vi "Spark MAX_Extract out all Parameter Data.vi"(11 "MotorControlDeviceRef":T4={"DeviceStatus"={"status"=FALSE, "code"=0, "source"=""}, "Type"=enum."CAN", "PWM"={"PWM Channel"=enum."Invalid", "DeadBand"={"Name"="", "maxPositivePwm"=0, "minPositivePwm"=0, "centerPwm"=0, "maxNegativePwm"=0, "minNegativePwm"=0, "angularRange"=0}}, "CAN"={"Device Number"=8, "SetOutput VI Ref"=variant, "GetOutput VI Ref"=variant, "Enable VI Ref"=variant, "Disable VI Ref"=variant, "Data"=variant(cluster{"Ext ID":u32, "Motor Type":enum16{"Brushed", "Brushless"}} {"Ext ID"=33882120, "Motor Type"=enum."Brushed"})}, "Invert"=FALSE, "DIO PWM"={"PWM \"Enable\" Channel"=enum."Invalid", "DIOChannel"=enum."Invalid", "PWM Rate"=0.0}}) -> (0 "Error Out":errorcluster, 1 "Type Out":T3, 2 "Raw Parameter Out":u32, 3 "MotorControlDeviceRef Out":T4={"DeviceStatus"={"status"=FALSE, "code"=0, "source"=""}, "Type"=enum."CAN", "PWM"={"PWM Channel"=enum."Invalid", "DeadBand"={"Name"="", "maxPositivePwm"=0, "minPositivePwm"=0, "centerPwm"=0, "maxNegativePwm"=0, "minNegativePwm"=0, "angularRange"=0}}, "CAN"={"Device Number"=8, "SetOutput VI Ref"=variant, "GetOutput VI Ref"=variant, "Enable VI Ref"=variant, "Disable VI Ref"=variant, "Data"=variant(cluster{"Ext ID":u32, "Motor Type":enum16{"Brushed", "Brushless"}} {"Ext ID"=33882120, "Motor Type"=enum."Brushed"})}, "Invert"=FALSE, "DIO PWM"={"PWM \"Enable\" Channel"=enum."Invalid", "DIOChannel"=enum."Invalid", "PWM Rate"=0.0}}, 5 "Array Out":T1[](array[typedef]) {"Float" format="%#_4f"})   [LabVIEW 2020]
uses:
  <vilib>/Rock Robotics/WPI/MotorControl/WPI_MotorControlDeviceRef.ctl
  <vilib>/Rock Robotics/WPI/MotorControl/WPI_MotorControlType.ctl
  <vilib>/Rock Robotics/SystemInterfaces/DIO/FPGA_DIOPWMChannel.ctl
  <vilib>/Rock Robotics/WPI/PWM/WPI_PWMDeadband.ctl
  <vilib>/Rock Robotics/SystemInterfaces/DIO/FPGA_DIOChannel.ctl
  <vilib>/Rock Robotics/WPI/ThirdParty/REV Robotics/REVLib/Typedef/Spark MAX Parameter Type.ctl
  Cluster_Spark Max parameter data.ctl
  <vilib>/Rock Robotics/WPI/ThirdParty/REV Robotics/REVLib/Typedef/Spark MAX Parameter ID.ctl
  <vilib>/Rock Robotics/WPI/ThirdParty/REV Robotics/REVLib/Typedef/Spark MAX Variant Data.ctl
  7c812163-354c-4a87-889c-090e08b6996c.vi
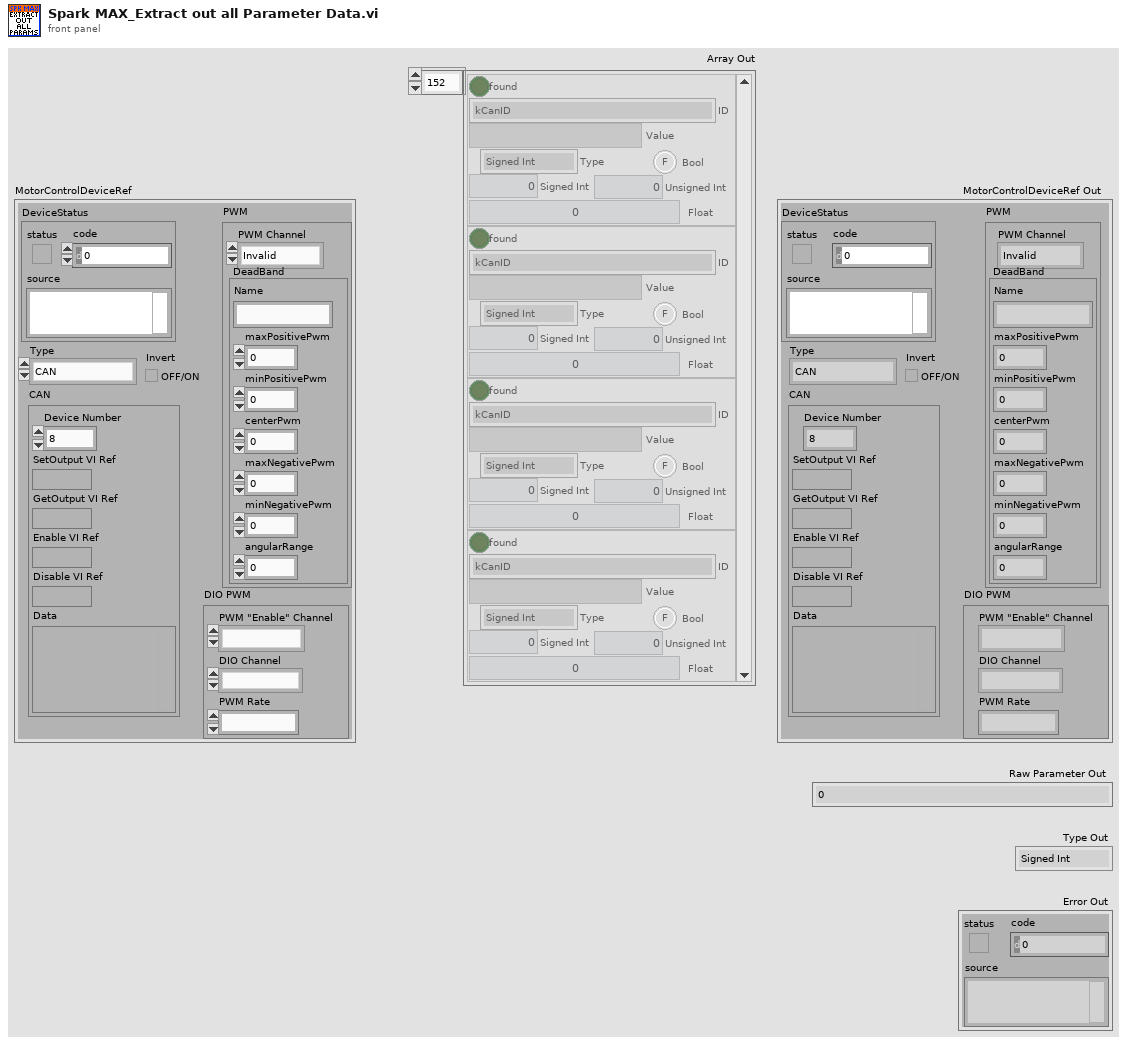
[diagram p1: front panel]
types:
  T1 = typedef "Cluster_Spark Max parameter data.ctl" = cluster{"found":bool, "ID":T2, "Value":string, "Type":T3, "Signed Int":i32, "Unsigned Int":u32, "Float":dbl, "Bool":bool}
  T2 = typedef "Spark MAX Parameter ID.ctl" = enum16{"kCanID", "kInputMode", "kMotorType", "kCommAdvance", "kSensorType", "kCtrlType", "kIdleMode", "kInputDeadband", "kFeedbackSensorPID0", "kFeedbackSensorPID1", "kPolePairs", "kCurrentChop", "kCurrentChopCycles", "kP_0", "kI_0", "kD_0", "kF_0", "kIZone_0", "kDFilter_0", "kOutputMin_0", "kOutputMax_0", "kP_1", "kI_1", "kD_1", "kF_1", "kIZone_1", "kDFilter_1", "kOutputMin_1", "kOutputMax_1", "kP_2", "kI_2", "kD_2", "kF_2", "kIZone_2", "kDFilter_2", "kOutputMin_2", "kOutputMax_2", "kP_3", "kI_3", "kD_3", "kF_3", "kIZone_3", "kDFilter_3", "kOutputMin_3", "kOutputMax_3", "kInverted", "kOutputRatio", "kSerialNumberLow", "kSerialNumberMid", "kSerialNumberHigh", "kLimitSwitchFwdPolarity", "kLimitSwitchRevPolarity", "kHardLimitFwdEn", "kHardLimitRevEn", "kSoftLimitFwdEn", "kSoftLimitRevEn", "kRampRate", "kFollowerID", "kFollowerConfig", "kSmartCurrentStallLimit", "kSmartCurrentFreeLimit", "kSmartCurrentConfig", "kSmartCurrentReserved", "kMotorKv", "kMotorR", "kMotorL", "kMotorRsvd1", "kMotorRsvd2", "kMotorRsvd3", "kEncoderCountsPerRev", "kEncoderAverageDepth", "kEncoderSampleDelta", "kEncoderInverted", "kEncoderRsvd1", "kClosedLoopVoltageMode", "kCompensatedNominalVoltage", "kSmartMotionMaxVelocity_0", "kSmartMotionMaxAccel_0", "kSmartMotionMinVelOutput_0", "kSmartMotionAllowedClosedLoopError_0", "kSmartMotionAccelStrategy_0", "kSmartMotionMaxVelocity_1", "kSmartMotionMaxAccel_1", "kSmartMotionMinVelOutput_1", "kSmartMotionAllowedClosedLoopError_1", "kSmartMotionAccelStrategy_1", "kSmartMotionMaxVelocity_2", "kSmartMotionMaxAccel_2", "kSmartMotionMinVelOutput_2", "kSmartMotionAllowedClosedLoopError_2", "kSmartMotionAccelStrategy_2", "kSmartMotionMaxVelocity_3", "kSmartMotionMaxAccel_3", "kSmartMotionMinVelOutput_3", "kSmartMotionAllowedClosedLoopError_3", "kSmartMotionAccelStrategy_3", "kIMaxAccum_0", "kSlot3Placeholder1_0", "kSlot3Placeholder2_0", "kSlot3Placeholder3_0", "kIMaxAccum_1", "kSlot3Placeholder1_1", "kSlot3Placeholder2_1", "kSlot3Placeholder3_1", "kIMaxAccum_2", "kSlot3Placeholder1_2", "kSlot3Placeholder2_2", "kSlot3Placeholder3_2", "kIMaxAccum_3", "kSlot3Placeholder1_3", "kSlot3Placeholder2_3", "kSlot3Placeholder3_3", "kPositionConversionFactor", "kVelocityConversionFactor", "kClosedLoopRampRate", "kSoftLimitFwd", "kSoftLimitRev", "kSoftLimitRsvd0", "kSoftLimitRsvd1", "kAnalogPositionConversion", "kAnalogVelocityConversion", "kAnalogAverageDepth", "kAnalogSensorMode", "kAnalogInverted", "kAnalogSampleDelta", "kAnalogRsvd0", "kAnalogRsvd1", "kDataPortConfig", "kAltEncoderCountsPerRev", "kAltEncoderAverageDepth", "kAltEncoderSampleDelta", "kAltEncoderInverted", "kAltEncoderPositionConversion", "kAltEncoderVelocityConversion", "kAltEncoderRsvd0", "kAltEncoderRsvd1", "kHallSensorSampleRate", "kHallSensorAverageDepth", "kNumParameters", "kDutyCyclePositionFactor", "kDutyCycleVelocityFactor", "kDutyCycleInverted", "kDutyCycleSensorMode", "kDutyCycleAverageDepth", "kDutyCycleSampleDelta", "kDutyCycleOffsetv1p6p2", "kDutyCycleRsvd0", "kDutyCycleRsvd1", "kDutyCycleRsvd2", "kPositionPIDWrapEnable", "kPositionPIDMinInput", "kPositionPIDMaxInput", "kDutyCycleZeroCentered", "kDutyCyclePrescalar", "kDutyCycleOffset"}
  T3 = typedef "Spark MAX Parameter Type.ctl" = enum16{"Signed Int", "Unsigned Int", "Float", "Bool"}
  T4 = typedef "WPI_MotorControlDeviceRef.ctl" = cluster{"DeviceStatus":errorcluster, "Type":T5, "PWM":cluster{"PWM Channel":T6, "DeadBand":T7}, "CAN":cluster{"Device Number":u8, "SetOutput VI Ref":variant, "GetOutput VI Ref":variant, "Enable VI Ref":variant, "Disable VI Ref":variant, "Data":variant}, "Invert":bool, "DIO PWM":cluster{"PWM \"Enable\" Channel":T6, "DIOChannel":T8, "PWM Rate":dbl}}
  T5 = typedef "WPI_MotorControlType.ctl" = enum16{"PWM", "CAN", "DIO PWM"}
  T6 = typedef "FPGA_DIOPWMChannel.ctl" = enum8{"PWM 0", "PWM 1", "PWM 2", "PWM 3", "PWM 4", "PWM 5", "PWM 6", "PWM 7", "PWM 8", "PWM 9", "PWM MXP 0", "PWM MXP 1", "PWM MXP 2", "PWM MXP 3", "PWM MXP 4", "PWM MXP 5", "PWM MXP 6", "PWM MXP 7", "PWM MXP 8", "PWM MXP 9", "Invalid"}
  T7 = typedef "WPI_PWMDeadband.ctl" = cluster{"Name":string, "maxPositivePwm":i32, "minPositivePwm":i32, "centerPwm":i32, "maxNegativePwm":i32, "minNegativePwm":i32, "angularRange":u16}
  T8 = typedef "FPGA_DIOChannel.ctl" = enum8{"DIO 0", "DIO 1", "DIO 2", "DIO 3", "DIO 4", "DIO 5", "DIO 6", "DIO 7", "DIO 8", "DIO 9", "DIO MXP 0", "DIO MXP 1", "DIO MXP 2", "DIO MXP 3", "DIO MXP 4", "DIO MXP 5", "DIO MXP 6", "DIO MXP 7", "DIO MXP 8", "DIO MXP 9", "DIO MXP 10", "DIO MXP 11", "DIO MXP 12", "DIO MXP 13", "DIO MXP 14", "DIO MXP 15", "SPI Port CS1", "SPI Port CS2", "SPI Port CS3", "SPI Port MISO", "SPI Port MOSI", "Invalid"}
  T9 = typedef "Spark MAX Variant Data.ctl" = cluster{"Ext ID":u32, "Status 0 Session Handle":u32, "Status 1 Session Handle":u32, "Param Session Handle":u32, "Param Cache ref":refnum<data-value>, "CAN Timeout":u32, "Status 2 Session Handle":u32, "Status 3 Session Handle":u32, "Inverted No WPILib":bool, "Has Configured Limit Sw":bool, "Has Configured Alt Encoder":bool, "Status 4 Session Handle":u32}
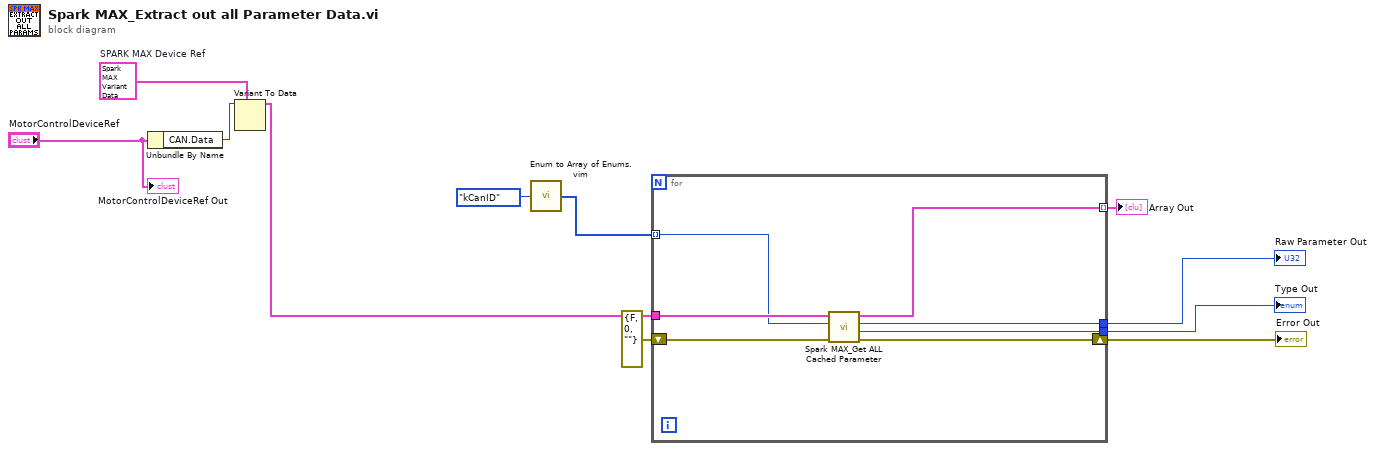
[diagram p0: block diagram]
diagram:
  w10 = T9 {"Ext ID"=0, "Status 0 Session Handle"=0, "Status 1 Session Handle"=0, "Param Session Handle"=0, "Param Cache ref"=refnum, "CAN Timeout"=0, "Status 2 Session Handle"=0, "Status 3 Session Handle"=0, "Inverted No WPILib"=FALSE, "Has Configured Limit Sw"=FALSE, "Has Configured Alt Encoder"=FALSE, "Status 4 Session Handle"=0}  # SPARK MAX Device Ref
  n1 = Unbundle By Name("MotorControlDeviceRef") -> ("CAN.Data"=w11:variant)
  n2 = Variant To Data(type=w10, Variant=w11) -> (data=w2:T9)  [unwired: 1 in, 1 out]
  n3 = call "Enum to Array of Enums.vim"("enum"=Spark_MAX_Parameter_ID."kCanID" ("Parameter ID")) -> ("array of enums"=w3:T2[])
  n4 = for {
    tunnel: w2 -> [w18]
    tunnel: [w17] -> w8
    tunnel: [w16] -> w7
    tunnel: w3 -> [w13] mode=indexing
    shift-right: [w15] -> w6
    shift-left: errorcluster {"status"=FALSE, "code"=0, "source"=""} ("error out") -> [w14]
    tunnel: [w12] -> w5 mode=indexing
    n5 = call "Spark MAX_Get ALL Cached Parameter.vi"("error in (no error)"=w14, "Parameter ID"=w13, "SPARK MAX Device Ref in"=w18) -> ("error out"=w15:errorcluster, "Parameter Type"=w16:T3, "Parameter Raw"=w17:u32, "output cluster"=w12:T1)  [unwired: 4 in, 1 out]
  }
  "Error Out" <- w6
  "Raw Parameter Out" <- w8
  "Type Out" <- w7
  "Array Out" <- w5
  "MotorControlDeviceRef Out" <- "MotorControlDeviceRef"
